vi "produceTimingTicks.vi"(8 "error in (no error)":errorcluster, 10 "Channel":refnum<class "Channel.lvclass">, 11 "device in":refnum<class "device.lvclass">) -> (0 "error out":errorcluster, 3 "device out":refnum<class "device.lvclass">)   [LabVIEW 2011, in "Tools.lvlib" / "DatabaseHelpers.lvlib" / "device.lvclass"]
uses:
  device.lvclass
  Channel/Channel.lvclass
  device.lvclass/device.ctl
  Scripting/ScriptingEvent/ScriptEventList/ScriptEventList.lvclass
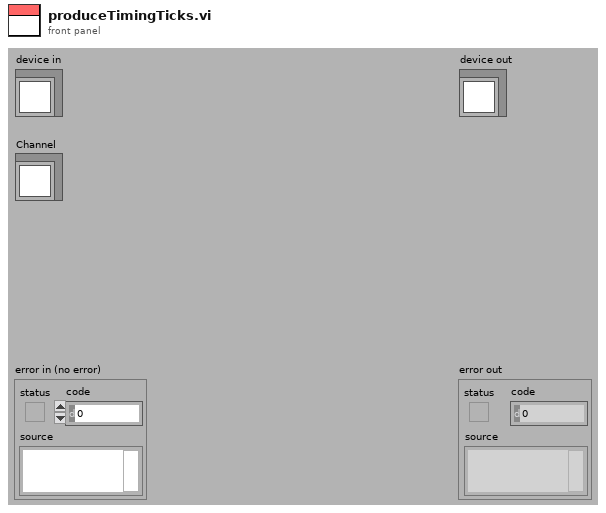
[diagram p1: front panel]
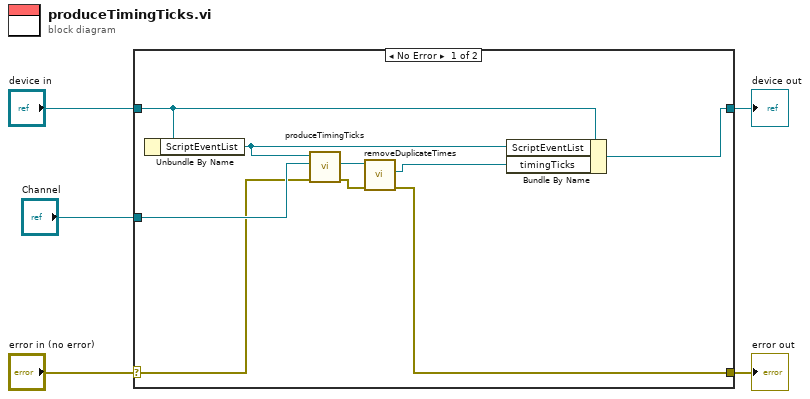
[diagram p0: block diagram]
diagram:
  n1 = case shown="No Error" "error in (no error)" {
    selector: "error in (no error)" -> [w10 w16]
    tunnel: [w7 w16] -> w4
    tunnel: [w12 w15] -> w2
    tunnel: "device in" -> [w13 w15]
    tunnel: "Channel" -> [w14 _]
    frame No Error {
      n2 = Unbundle By Name(w13) -> ("ScriptEventList"=w11:refnum<class "ScriptEventList.lvclass">)
      n3 = call-dynamic "produceTimingTicks.vi"("error in (no error)"=w10, "Channel"=w14, "ScriptEventList in"=w11) -> ("error out"=w8:errorcluster, "timingTickList"=w9:refnum<class "ScriptEventList.lvclass">)  [unwired: 6 in, 1 out]
      n4 = call "removeDuplicateTimes.vi"("error in (no error)"=w8, "ScriptEventList in"=w9) -> ("error out"=w7:errorcluster, "list"=w6:refnum<class "ScriptEventList.lvclass">)  [unwired: 7 in, 1 out]
      n5 = Bundle By Name(cluster=w13, "ScriptEventList"=w11, "timingTicks"=w6) -> (w12:refnum<class "device.lvclass">)
    }
    frame Error {
    }
  }
  "error out" <- w4
  "device out" <- w2
